vi "FL Create Antecedent.vi"(8 "error in (no error)":errorcluster, 9 "condition":T2 items=["=", "!="], 10 "membership function index":i32, 11 "variable index":i32) -> (0 "error out":errorcluster, 3 "antecedent":T1 {"Var Index" min=0; "Cond" items=["=", "!="]; "MF Index" min=0})   [LabVIEW 2017, in "NI_Fuzzy_Logic_API.lvlib"]
doc: "Creates an antecedent, or IF portion, of a rule for a fuzzy system. An antecedent consists of three parts: an input linguistic variable, an operator that specifies whether to calculate the degree of membership or the degree of non-membership of the input linguistic variable within a linguistic term, and a linguistic term.\n\nYou can use the Build Array function or a loop to build an array of rule antecedents that you create with this VI. You then can wire the array to the <B>antecedents</B> input of the FL Create Rule VI."
uses:
  <vilib>/addons/Fuzzy Logic/NI_Fuzzy_Logic_API.lvlib
  <vilib>/addons/Fuzzy Logic/TypeDefs/FL Modifier.ctl
  <vilib>/addons/Fuzzy Logic/TypeDefs/FL Antecedent.ctl
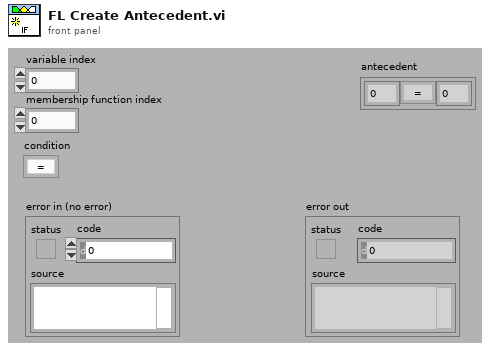
[diagram p1: front panel]
types:
  T1 = typedef "NI_Fuzzy_Logic_API.lvlib/FL Antecedent.ctl" = cluster{"Var Index":i32, "MF Index":i32, "Cond":T2}
  T2 = typedef "NI_Fuzzy_Logic_API.lvlib/FL Modifier.ctl" = u16
  T3 = cluster{"variable index":i32, "membership function index":i32, "condition":T2}
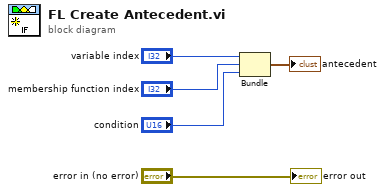
[diagram p0: block diagram]
diagram:
  n1 = Bundle("variable index"="variable index", "membership function index"="membership function index", "condition"="condition") -> (→"antecedent":T3)  [unwired: 1 out]
  "error out" <- "error in (no error)"
